vi "FestoCPX.booleanToFrame.vi"(10 "Raw Array":bool[](array[boolean])) -> (2 "Bytes DO":u16[](array[numeric]) format="%04x")   [LabVIEW 2014]
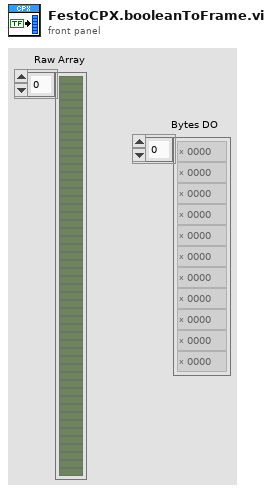
[diagram p1: front panel]
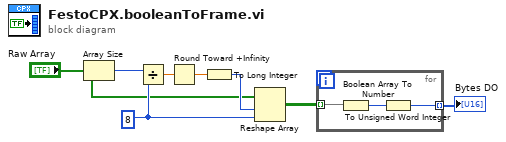
[diagram p0: block diagram]
diagram:
  w5 = 8 ("dimension size")
  n1 = Array Size(array="Raw Array") -> (size(s)=w6:i32)
  n2 = Divide(x=w6, y=w5) -> (x/y=w7:dbl)
  n3 = Round Toward +Infinity(x=w7) -> (ceil(x): smallest int >= x=w8:dbl)
  n4 = To Long Integer(number=w8) -> (32bit integer=w4:i32)
  n5 = Reshape Array("Raw Array", w4, w5) -> (w3:bool[][])
  n6 = for {
    tunnel: w3 -> [w11] mode=indexing
    tunnel: [w9] -> w1 mode=indexing
    n7 = Boolean Array To Number(Boolean array=w11) -> (number=w10:u32)
    n8 = To Unsigned Word Integer(number=w10) -> (unsigned 16bit integer=w9:u16)
  }
  "Bytes DO" <- w1
